vi "全局变量.vi"() -> ()   [LabVIEW 2011]
panel:
  in  "Counts":u16
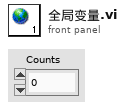
[diagram p1: front panel]
diagram:
